vi "Wait on Disconnect.vi"(8 "error in (no error)":errorcluster, 11 "TCP Client in":refnum<class "TCP Client.lvclass">) -> (0 "error out":errorcluster, 3 "TCP Client out":refnum<class "TCP Client.lvclass">)   [LabVIEW 2020, in "Stream-TCP.lvlib" / "TCP Client.lvclass"]
uses:
  TCP Client.lvclass
  C:/dev/lv20CE/relink/lv-stream/stream/Connection/Connection.lvclass
  lv-stream/stream/Connection/State.ctl
  Client Command.ctl
  Stream-TCP.lvlib
  lv-stream/stream/Connection/Connection.lvclass
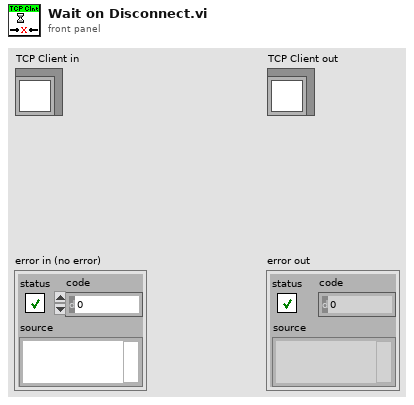
[diagram p1: front panel]
types:
  T1 = typedef "Stream.lvlib/Connection.lvclass/State.ctl" = enum16{"Closed", "Idle", "Connecting", "Connected", "Shutdown"}
  T2 = typedef "Stream-TCP.lvlib/Client Command.ctl" = enum16{"Connect", "Close", "Shutdown", "Reconnect"}
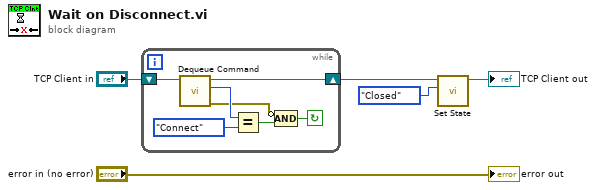
[diagram p0: block diagram]
diagram:
  n1 = while {
    shift-right: [w6] -> w3
    shift-left: "TCP Client in" -> [w12]
    stop <- w7 continue-if-true
    n2 = call "Dequeue Command.vi"("TCP Client in"=w12) -> ("error out"=w8:errorcluster, "Command"=w11:T2, "TCP Client out"=w6:refnum<class "TCP Client.lvclass">)  [unwired: 7 in, 1 out]
    n3 = Equal?(x=w11, y=Client_Command."Connect") -> (x = y?=w9:bool)
    n4 = Compound Arithmetic op=AND(invert w8, w9) -> (w7:bool)
  }
  n5 = call "Set State.vi"("State"=State."Closed", "Connection in"=w3) -> ("Connection out"=→"TCP Client out":refnum<class "TCP Client.lvclass">)  [unwired: 8 in, 1 out]
  "error out" <- "error in (no error)"
